vi "Load Configs.vi"(8 "error in":errorcluster) -> (0 "error out":errorcluster)   [LabVIEW 2011]
uses:
  Global Coude.vi
  <vilib>/Utility/config.llb/NI_LVConfig.lvlib
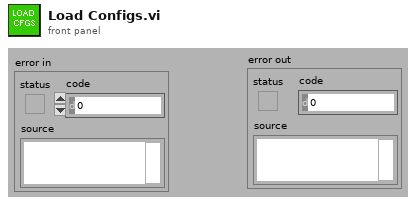
[diagram p1: front panel]
types:
  T1 = cluster{"Mec ID":string, "VISA Mec":refnum<visa-resource-name>, "Mec PosLimit":string, "Mec NegLimit":string, "Mec Factor":dbl, "Mec Speed":dbl, "Mec Acceleration":dbl, "MecOffset":string, "MecTargets":dbl[], "MecEnabled":bool, "Mec Target":dbl}
  T2 = typedef "NI_LVConfig.lvlib/Config Data RefNum.ctl" = refnum<k1>
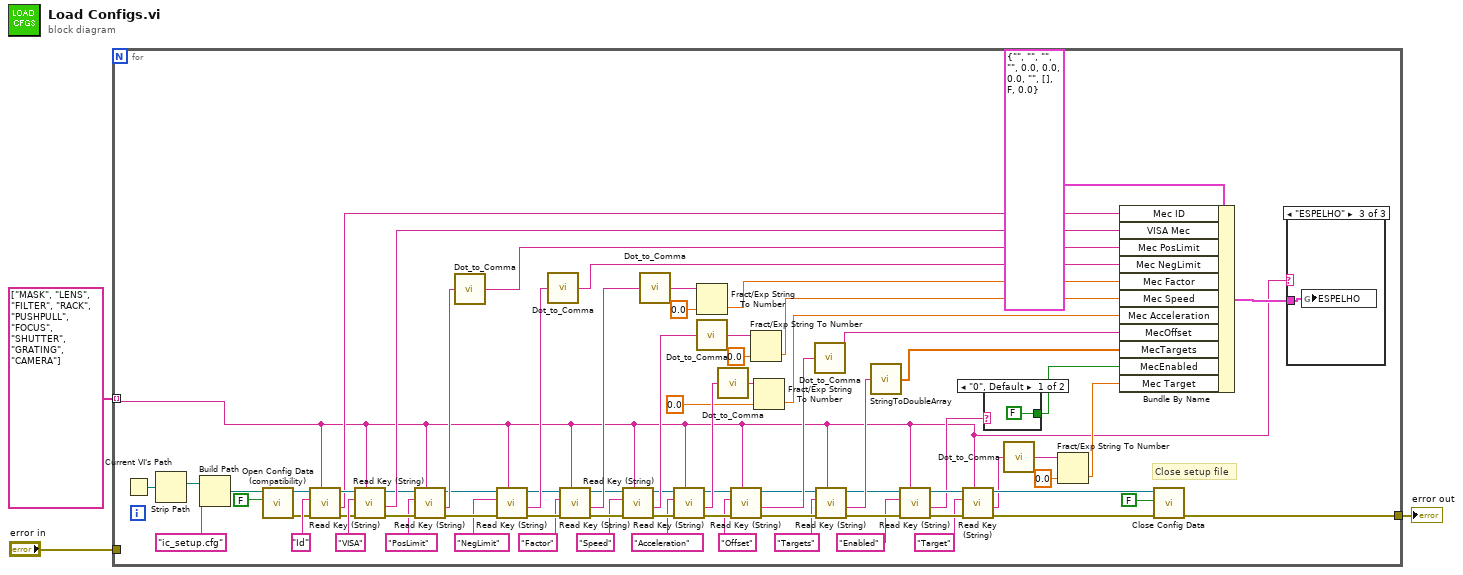
[diagram p0: block diagram]
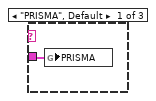
[diagram p2: hidden frame]
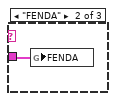
[diagram p3: hidden frame]
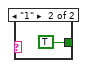
[diagram p4: hidden frame]
diagram:
  n1 = for {
    tunnel: string[] ["MASK", "LENS", "FILTER", "RACK", "PUSHPULL", "FOCUS", "SHUTTER", "GRATING", "CAMERA"] -> [w4] mode=indexing
    tunnel: [w7] -> w2
    tunnel: "error in" -> [_]
    # "Close setup file"
    n2 = Current VI's Path() -> (path=w30:path)
    n3 = Strip Path(path=w30) -> (stripped path=w31:path)  [unwired: 1 out]
    n4 = Build Path(base path=w31, name or relative path="ic_setup.cfg") -> (appended path=w11:path)
    n5 = call <vilib>:"Open Config Data (compatibility).vi"("create file if necessary (T)"=FALSE ("create file if necessary? (T)"), "configuration file path"=w11) -> ("error out"=w9:errorcluster, "refnum"=w8:T2)  [unwired: 7 in, 1 out]
    n6 = call <vilib>:"Read Key (String).vi"("section"=w4, "error in (no error)"=w9, "key"="Id", "refnum"=w8) -> ("error out"=w13:errorcluster, "value"=w12:string, "refnum out"=w14:T2)  [unwired: 2 in, 3 out]
    n7 = call <vilib>:"Read Key (String).vi"("section"=w4, "error in (no error)"=w13, "key"="VISA", "refnum"=w14) -> ("error out"=w55:errorcluster, "value"=w69:string, "refnum out"=w51:T2)  [unwired: 2 in, 3 out]
    n8 = call <vilib>:"Read Key (String).vi"("section"=w4, "error in (no error)"=w55, "key"="PosLimit", "refnum"=w51) -> ("error out"=w57:errorcluster, "value"=w61:string, "refnum out"=w56:T2)  [unwired: 2 in, 3 out]
    n9 = call "Dot_to_Comma.vi"("String in"=w61) -> ("String out"=w70:string)
    n10 = call <vilib>:"Read Key (String).vi"("section"=w4, "error in (no error)"=w57, "key"="NegLimit", "refnum"=w56) -> ("error out"=w54:errorcluster, "value"=w62:string, "refnum out"=w50:T2)  [unwired: 2 in, 3 out]
    n11 = call "Dot_to_Comma.vi"("String in"=w62) -> ("String out"=w71:string)
    n12 = call <vilib>:"Read Key (String).vi"("section"=w4, "error in (no error)"=w54, "key"="Factor", "refnum"=w50) -> ("error out"=w53:errorcluster, "value"=w63:string, "refnum out"=w49:T2)  [unwired: 2 in, 3 out]
    n13 = call <vilib>:"Read Key (String).vi"("section"=w4, "error in (no error)"=w53, "key"="Speed", "refnum"=w49) -> ("error out"=w52:errorcluster, "value"=w59:string, "refnum out"=w48:T2)  [unwired: 2 in, 3 out]
    n14 = call "Dot_to_Comma.vi"("String in"=w63) -> ("String out"=w64:string)
    n15 = call <vilib>:"Read Key (String).vi"("section"=w4, "error in (no error)"=w52, "key"="Acceleration", "refnum"=w48) -> ("error out"=w43:errorcluster, "value"=w65:string, "refnum out"=w42:T2)  [unwired: 2 in, 3 out]
    n16 = Fract/Exp String To Number(string=w64, default (0 dbl)=0.0 ("default (0 DBL)")) -> (number=w72:dbl)  [unwired: 3 out]
    n17 = call "Dot_to_Comma.vi"("String in"=w59) -> ("String out"=w60:string)
    n18 = call "Dot_to_Comma.vi"("String in"=w65) -> ("String out"=w66:string)
    n19 = call <vilib>:"Read Key (String).vi"("section"=w4, "error in (no error)"=w43, "key"="Offset", "refnum"=w42) -> ("error out"=w41:errorcluster, "value"=w67:string, "refnum out"=w40:T2)  [unwired: 2 in, 3 out]
    n20 = Fract/Exp String To Number(string=w60, default (0 dbl)=0.0) -> (number=w73:dbl)  [unwired: 3 out]
    n21 = Fract/Exp String To Number(string=w66, default (0 dbl)=0.0) -> (number=w74:dbl)  [unwired: 3 out]
    n22 = call "Dot_to_Comma.vi"("String in"=w67) -> ("String out"=w75:string)
    n23 = call <vilib>:"Read Key (String).vi"("section"=w4, "error in (no error)"=w41, "key"="Targets", "refnum"=w40) -> ("error out"=w26:errorcluster, "value"=w33:string, "refnum out"=w29:T2)  [unwired: 2 in, 3 out]
    n24 = call "StringToDoubleArray.vi"("String"=w33) -> ("MecTargets"=w76:dbl[])
    n25 = call <vilib>:"Read Key (String).vi"("section"=w4, "error in (no error)"=w26, "key"="Enabled", "refnum"=w29) -> ("error out"=w25:errorcluster, "value"=w21:string, "refnum out"=w28:T2)  [unwired: 2 in, 3 out]
    n26 = call <vilib>:"Read Key (String).vi"("section"=w4, "error in (no error)"=w25, "key"="Target", "refnum"=w28) -> ("error out"=w24:errorcluster, "value"=w17:string, "refnum out"=w27:T2)  [unwired: 2 in, 3 out]
    n27 = case shown="\"0\", Default" w21 {
      tunnel: [FALSE TRUE] -> w20
      frame "0", Default {
      }
      frame "1" {
      }
    }
    n28 = call "Dot_to_Comma.vi"("String in"=w17) -> ("String out"=w19:string)
    n29 = Fract/Exp String To Number(string=w19, default (0 dbl)=0.0) -> (number=w16:dbl)  [unwired: 3 out]
    n30 = Bundle By Name(cluster=T1 {"Mec ID"="", "VISA Mec"="", "Mec PosLimit"="", "Mec NegLimit"="", "Mec Factor"=0.0, "Mec Speed"=0.0, "Mec Acceleration"=0.0, "MecOffset"="", "MecTargets"=[], "MecEnabled"=FALSE, "Mec Target"=0.0} ("CAM"), "Mec ID"=w12, "VISA Mec"=w69, "Mec PosLimit"=w70, "Mec NegLimit"=w71, "Mec Factor"=w72, "Mec Speed"=w73, "Mec Acceleration"=w74, "MecOffset"=w75, "MecTargets"=w76, "MecEnabled"=w20, "Mec Target"=w16) -> (w6:T1)
    n31 = call <vilib>:"Close Config Data.vi"("error in (no error)"=w24, "write file if changed (T)"=FALSE ("create file if necessary? (T)"), "refnum"=w27) -> ("error out"=w7:errorcluster)  [unwired: 8 out]
    n32 = case shown="\"ESPELHO\"" w4 {
      tunnel: w6 -> [w77 w78 w79]
      frame "PRISMA", Default {
        n33 = global write "Global Coude.vi" "PRISMA"(w77) -> ()
      }
      frame "FENDA" {
        n34 = global write "Global Coude.vi" "FENDA"(w78) -> ()
      }
      frame "ESPELHO" {
        n35 = global write "Global Coude.vi" "ESPELHO"(w79) -> ()
      }
    }
  }
  "error out" <- w2
